vi "CRC16.vi"(0 "DATA":string) -> (1 "CRC =":u32 format="%x", 2 "CRC-16":string)   [LabVIEW 2018]
panel:
  # "Polynom X16+X12+X5+1"
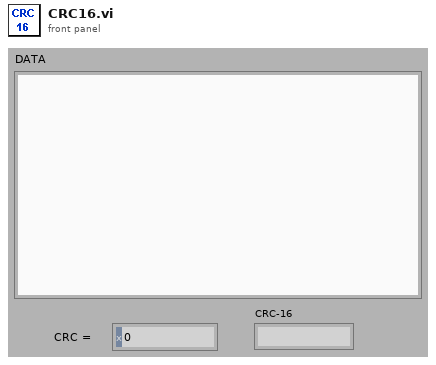
[diagram p1: front panel]
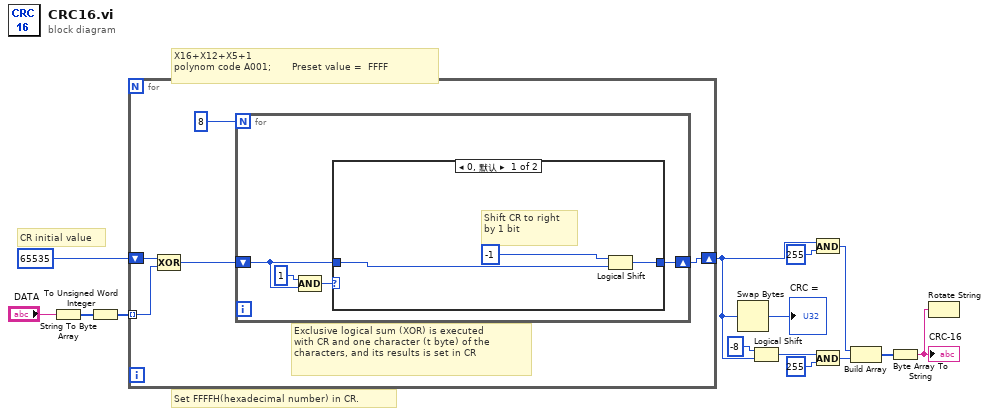
[diagram p0: block diagram]
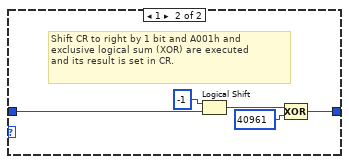
[diagram p2: hidden frame]
diagram:
  # "Set FFFFH(hexadecimal number) in CR."
  # "CR initial value"
  # "X16+X12+X5+1\npolynom code A001;       Preset value =  FFFF"
  n1 = String To Byte Array(string="DATA") -> (unsigned byte array=w13:u8[])
  n2 = To Unsigned Word Integer(number=w13) -> (unsigned 16bit integer=w12:u16[])
  n3 = for {
    shift-right: [w16] -> w6
    shift-left: u16 65535 -> [w17]
    tunnel: w12 -> [w15] mode=indexing
    # "Exclusive logical sum (XOR) is executed\nwith CR and one character (t byte) of the\ncharacters, and its results is set in CR"
    n4 = Compound Arithmetic op=XOR(w17, w15) -> (w18:u32)
    n5 = for {
      N: 8 -> [_]
      shift-right: [w22] -> w16
      shift-left: w18 -> [w21]
      n6 = Compound Arithmetic op=AND(u16 1, w21) -> (w20:u32)
      n7 = case shown="0, 默认" w20 {
        tunnel: [w25 w30] -> w22
        tunnel: w21 -> [w24 w27]
        frame 0, Default {
          # "Shift CR to right\nby 1 bit"
          n8 = Logical Shift(y=i16 -1, x=w24) -> (x << y=w25:u32)
        }
        frame 1 {
          # "Shift CR to right by 1 bit and A001h and\nexclusive logical sum (XOR) are executed\nand its result is set in CR."
          n9 = Logical Shift(y=i16 -1, x=w27) -> (x << y=w29:u32)
          n10 = Compound Arithmetic op=XOR(w29, u32 40961) -> (w30:u32)
        }
      }
    }
  }
  n11 = Swap Bytes(anything=w6) -> (byte swapped=→"CRC =":u32)
  n12 = Logical Shift(y=i16 -8, x=w6) -> (x << y=w8:u32)
  n13 = And(x=w6, y=u16 255) -> (x .and. y?=w4:u32)
  n14 = And(x=w8, y=u16 255) -> (x .and. y?=w3:u32)
  n15 = Build Array(w4, w3) -> (w2:u32[])
  n16 = Byte Array To String(unsigned byte array=w2) -> (string=w1:string)
  "CRC-16" <- w1
  n17 = Rotate String(1:w1) -> ()  [unwired: 1 out]
